vi "test_ccd_xAxisConversionType.vi"(8 "error in":errorcluster, 11 "CCD in":refnum<class "CCD.lvclass">) -> (0 "error out":errorcluster, 3 "CCD out":refnum<class "CCD.lvclass">)   [LabVIEW 2023, in "horiba.test.lvlib"]
uses:
  horiba.test.lvlib
  Classes/CCD/CCD.lvclass
  C:/Projects/Horiba/horiba-labview-sdk/Source/Classes/GenericDevice/GenericDevice.lvclass
  <vilib>/addons/_JKI Toolkits/Caraya/classes/Assert/Assert Equal Value and Type_Variant.vi
  <vilib>/addons/_JKI Toolkits/Caraya/classes/Test/Test.lvclass
  <vilib>/addons/_JKI Toolkits/Caraya/classes/Assert/Assert.lvclass
  <userlib>/_OpenG.lib/lvdata/lvdata.llb/openg_variant.lvlib
panel:
  # "Connector Pane"
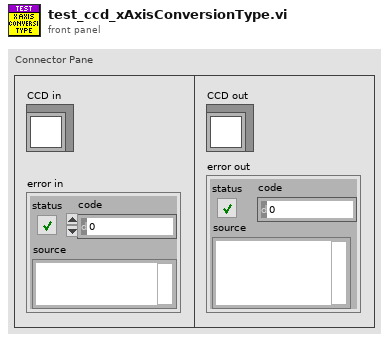
[diagram p1: front panel]
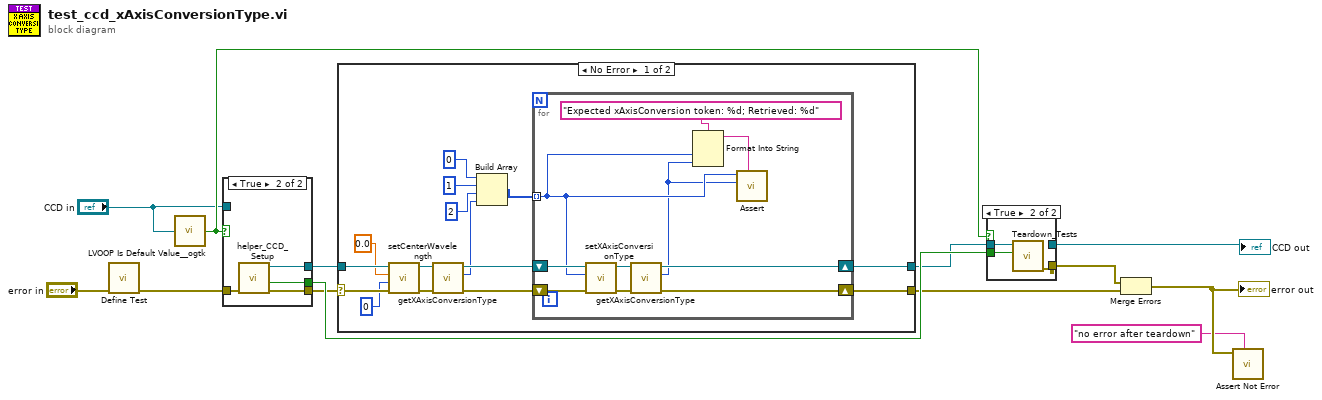
[diagram p0: block diagram]
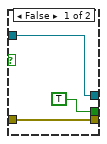
[diagram p3: hidden frame]
diagram:
  n1 = call <vilib>:"Define Test.vi"("error in (no error)"="error in") -> ("error out"=w8:errorcluster)  [unwired: 9 in, 1 out]
  n2 = call <userlib>:"LVOOP Is Default Value__ogtk.vi"("Object"="CCD in") -> ("Is Default Value?"=w9:bool)
  n3 = case shown="True" w9 {
    tunnel: w8 -> [w15 w20]
    tunnel: [w15 w19] -> w4
    tunnel: [w16 w18] -> w6
    tunnel: [TRUE ("Module Was Already Running?") w17] -> w10
    tunnel: "CCD in" -> [w16 _]
    frame False {
    }
    frame True {
      n4 = call "helper_CCD_Setup.vi"("error in"=w20) -> ("error out"=w19:errorcluster, "Module Was Already Running?"=w17:bool, "CCD out"=w18:refnum<class "CCD.lvclass">)  [unwired: 7 in, 1 out]
    }
  }
  n5 = case shown="No Error" w4 {
    selector: w4 -> [w35 w46]
    tunnel: [w33 w47] -> w5
    tunnel: w6 -> [w24 w47]
    tunnel: [w31 w46] -> w3
    frame No Error {
      n6 = call "setCenterWavelength.vi"("error in (no error)"=w35, "monoIndex"=0, "wavelength"=0.0, "CCD in"=w24) -> ("error out"=w25:errorcluster, "CCD out"=w23:refnum<class "CCD.lvclass">)  [unwired: 4 in, 2 out]
      n7 = call "getXAxisConversionType.vi"("error in (no error)"=w25, "CCD in"=w23) -> ("error out"=w32:errorcluster, "type"=w30:i32, "CCD out"=w34:refnum<class "CCD.lvclass">)  [unwired: 7 in]
      n8 = Build Array(0 ("element"), 1 ("element"), 2 ("element"), w30) -> (w29:i32[])
      n9 = for {
        shift-right: [w42] -> w33
        shift-left: w34 -> [w43]
        shift-right: [w40] -> w31
        shift-left: w32 -> [w41]
        tunnel: w29 -> [w37] mode=indexing
        n10 = call "setXAxisConversionType.vi"("error in (no error)"=w41, "type"=w37, "CCD in"=w43) -> ("error out"=w45:errorcluster, "CCD out"=w44:refnum<class "CCD.lvclass">)  [unwired: 5 in, 2 out]
        n11 = call "getXAxisConversionType.vi"("error in (no error)"=w45, "CCD in"=w44) -> ("error out"=w40:errorcluster, "type"=w36:i32, "CCD out"=w42:refnum<class "CCD.lvclass">)  [unwired: 7 in]
        n12 = Format Into String(format string="Expected xAxisConversion token: %d; Retrieved: %d", w37, w36) -> (resulting string=w39:string)  [unwired: 2 in, 1 out]
        n13 = call-poly <vilib>:"Assert.vi"("Label"=w39, "Y"=w36, "X"=w37) -> ()  [unwired: 7 in, 2 out]
      }
    }
    frame Error {
    }
  }
  n14 = case shown="True" w9 {
    tunnel: w5 -> [w48 w51]
    tunnel: [_ w50] -> w7
    tunnel: w10 -> [_ w49]
    tunnel: [w48 _] -> w1
    frame False {
    }
    frame True {
      n15 = call "Teardown_Tests.vi"("Module Was Already Running?"=w49, "horiba.lvlib:GenericDevice"=w51) -> ("error out"=w50:errorcluster)  [unwired: 8 in, 1 out]
    }
  }
  "CCD out" <- w1
  n16 = Merge Errors(w7, w3) -> (w12:errorcluster)
  "error out" <- w12
  n17 = call <vilib>:"Assert Not Error.vi"("Label"="no error after teardown", "Not Error?"=w12) -> ()  [unwired: 8 in, 2 out]
